vi "start_button_execution.vi"(8 "error in (no error)":errorcluster, 11 "control references":T1) -> (0 "error out":errorcluster, 1 "start?":bool, 2 "run mode":T2=enum."experiment mode")   [LabVIEW 2010]
uses:
  type_definitions/enumerations/run_mode_enum.ctl
  type_definitions/clusters/controls_refs.ctl
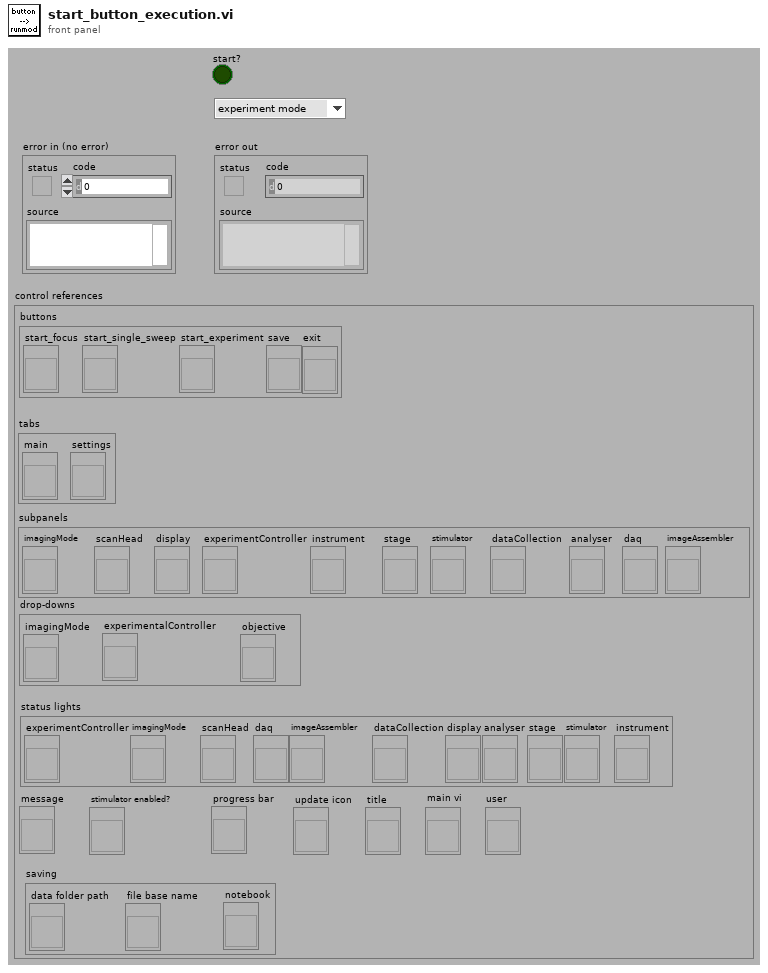
[diagram p1: front panel]
types:
  T1 = typedef "controls_refs.ctl" = cluster{"buttons":cluster{"start_focus":refnum<vi>, "start_single_sweep":refnum<vi>, "start_experiment":refnum<vi>, "save":refnum<vi>, "exit":refnum<vi>}, "tabs":cluster{"main":refnum<vi>, "settings":refnum<vi>}, "subpanels":cluster{"imagingMode":refnum<vi>, "scanHead":refnum<vi>, "display":refnum<vi>, "experimentController":refnum<vi>, "instrument":refnum<vi>, "stage":refnum<vi>, "stimulator":refnum<vi>, "dataCollection":refnum<vi>, "analyser":refnum<vi>, "daq":refnum<vi>, "imageAssembler":refnum<vi>}, "drop-downs":cluster{"imagingMode":refnum<vi>, "experimentalController":refnum<vi>, "objective":refnum<vi>}, "status lights":cluster{"experimentController":refnum<vi>, "imagingMode":refnum<vi>, "scanHead":refnum<vi>, "daq":refnum<vi>, "imageAssembler":refnum<vi>, "dataCollection":refnum<vi>, "display":refnum<vi>, "analyser":refnum<vi>, "stage":refnum<vi>, "stimulator":refnum<vi>, "instrument":refnum<vi>}, "message":refnum<vi>, "stimulator enabled?":refnum<vi>, "saving":cluster{"data folder path":refnum<vi>, "file base name":refnum<vi>, "notebook":refnum<vi>}, "progress bar":refnum<vi>, "update icon":refnum<vi>, "title":refnum<vi>, "main vi":refnum<vi>, "user":refnum<vi>}
  T2 = typedef "run_mode_enum.ctl" = enum16{"focus mode", "single sweep mode", "experiment mode"}
  T3 = enum8{"Enabled", "Disabled", "Disabled and Grayed Out"}
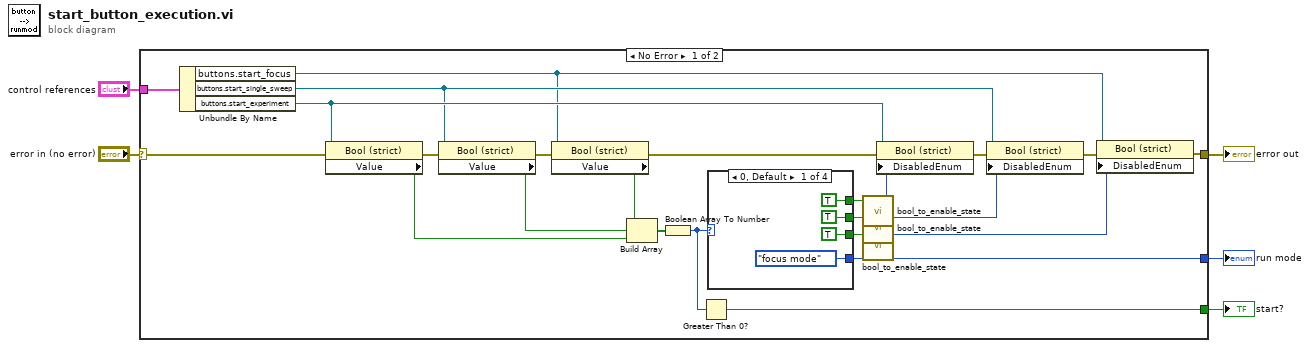
[diagram p0: block diagram]
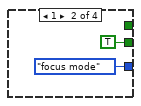
[diagram p2: hidden frame]
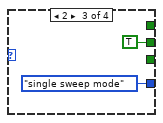
[diagram p3: hidden frame]
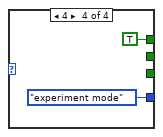
[diagram p4: hidden frame]
diagram:
  n1 = case shown="No Error" "error in (no error)" {
    selector: "error in (no error)" -> [w26 w40]
    tunnel: [w6 w40] -> w4
    tunnel: "control references" -> [w29 _]
    tunnel: [w21 _] -> w2
    tunnel: [w14 _] -> w1
    frame No Error {
      n2 = Unbundle By Name(w29) -> ("buttons.start_focus"=w16:refnum<vi>, "buttons.start_single_sweep"=w17:refnum<vi>, "buttons.start_experiment"=w19:refnum<vi>)
      n3 = property class="Bool (strict)"(reference=w19, error in=w26) -> (error out=w28:errorcluster, "Value"=w22:bool)  [unwired: 1 out]
      n4 = property class="Bool (strict)"(reference=w17, error in=w28) -> (error out=w27:errorcluster, "Value"=w23:bool)  [unwired: 1 out]
      n5 = property class="Bool (strict)"(reference=w16, error in=w27) -> (error out=w7:errorcluster, "Value"=w24:bool)  [unwired: 1 out]
      n6 = Build Array(w24, w23, w22) -> (w25:bool[])
      n7 = Boolean Array To Number(Boolean array=w25) -> (number=w20:u32)
      n8 = Greater Than 0?(x=w20) -> (x > 0?=w14:bool)
      n9 = case shown="0, Default" w20 {
        tunnel: [run_mode_enum."focus mode" ("run mode") run_mode_enum."focus mode" ("run mode") run_mode_enum."single sweep mode" ("run mode") run_mode_enum."experiment mode" ("run mode")] -> w21
        tunnel: [TRUE _ _ TRUE] -> w13
        tunnel: [TRUE _ TRUE _] -> w12
        tunnel: [TRUE TRUE _ _] -> w11
        frame 0, Default {
        }
        frame 1 {
        }
        frame 2 {
        }
        frame 4 {
        }
      }
      n10 = call "bool_to_enable_state.vi"("boolean in"=w13) -> ("enabled status out"=w10:T3)  [unwired: 4 in]
      n11 = call "bool_to_enable_state.vi"("boolean in"=w12) -> ("enabled status out"=w9:T3)  [unwired: 4 in]
      n12 = call "bool_to_enable_state.vi"("boolean in"=w11) -> ("enabled status out"=w8:T3)  [unwired: 4 in]
      n13 = property class="Bool (strict)"(reference=w19, error in=w7, "DisabledEnum"=w10) -> (error out=w15:errorcluster)  [unwired: 1 out]
      n14 = property class="Bool (strict)"(reference=w17, error in=w15, "DisabledEnum"=w9) -> (error out=w18:errorcluster)  [unwired: 1 out]
      n15 = property class="Bool (strict)"(reference=w16, error in=w18, "DisabledEnum"=w8) -> (error out=w6:errorcluster)  [unwired: 1 out]
    }
    frame Error {
    }
  }
  "error out" <- w4
  "run mode" <- w2
  "start?" <- w1
